vi "Camera Get Sensors.vi"(1 "Camera Global Data in":T1) -> (0 "Camera Global Data out":T1)   [LabVIEW 2013]
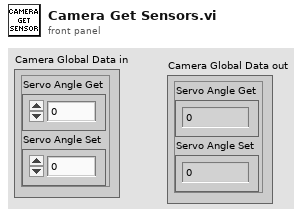
[diagram p1: front panel]
types:
  T1 = cluster{"Servo Angle Get":dbl, "Servo Angle Set":dbl}
  T2 = typedef "WPI_ServoDeviceRef.ctl" = cluster{"DeviceStatus":errorcluster, "Digital Module":T3, "PWM Channel":T4, "DeadBand":T5}
  T3 = typedef "FPGA_TypedefDigitalModule.ctl" = enum16{"Digital Module 1", "Digital Module 2"}
  T4 = typedef "FPGA_DIOPWMChannel.ctl" = enum8{"PWM 1", "PWM 2", "PWM 3", "PWM 4", "PWM 5", "PWM 6", "PWM 7", "PWM 8", "PWM 9", "PWM 10", "Invalid"}
  T5 = typedef "WPI_PWMDeadband.ctl" = cluster{"Name":string, "maxPositivePwm":i32, "minPositivePwm":i32, "centerPwm":i32, "maxNegativePwm":i32, "minNegativePwm":i32, "angularRange":u16}
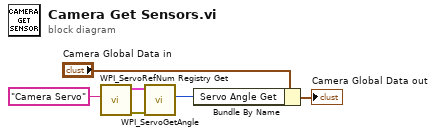
[diagram p0: block diagram]
diagram:
  n1 = call <vilib>:"WPI_ServoRefNum Registry Get.vi"("refnum name"="Camera Servo") -> ("error out"=w3:errorcluster, "ServoDeviceRef"=w4:T2)  [unwired: 9 in]
  n2 = call <vilib>:"WPI_ServoGetAngle.vi"("ServoDeviceRef"=w4, "error in (no error)"=w3) -> ("Angle"=w2:u16)  [unwired: 6 in, 2 out]
  n3 = Bundle By Name(cluster="Camera Global Data in", "Servo Angle Get"=w2) -> (→"Camera Global Data out":T1)
